vi "Lab3.vi"() -> ()   [LabVIEW 2021]
panel:
  in  "stop":bool
  out "Green 2":bool
  out "Yellow 2":bool
  out "Red 2":bool
  out "Green":bool
  out "Yellow":bool
  out "Red":bool
  out "Is it more than 5?":bool
  out "The number you input is:":string
  in  "Please input a number:":dbl
  in  "To Stop the Operation:":bool
  out "Condition":string
  out "Heater":bool
  out "Air Conditioner":bool
  out "Thermometer":dbl(slide) scale=0.0..100.0
  in  "Temperature":dbl
  # "Traffic Light 1"
  # "Traffic Light 2"
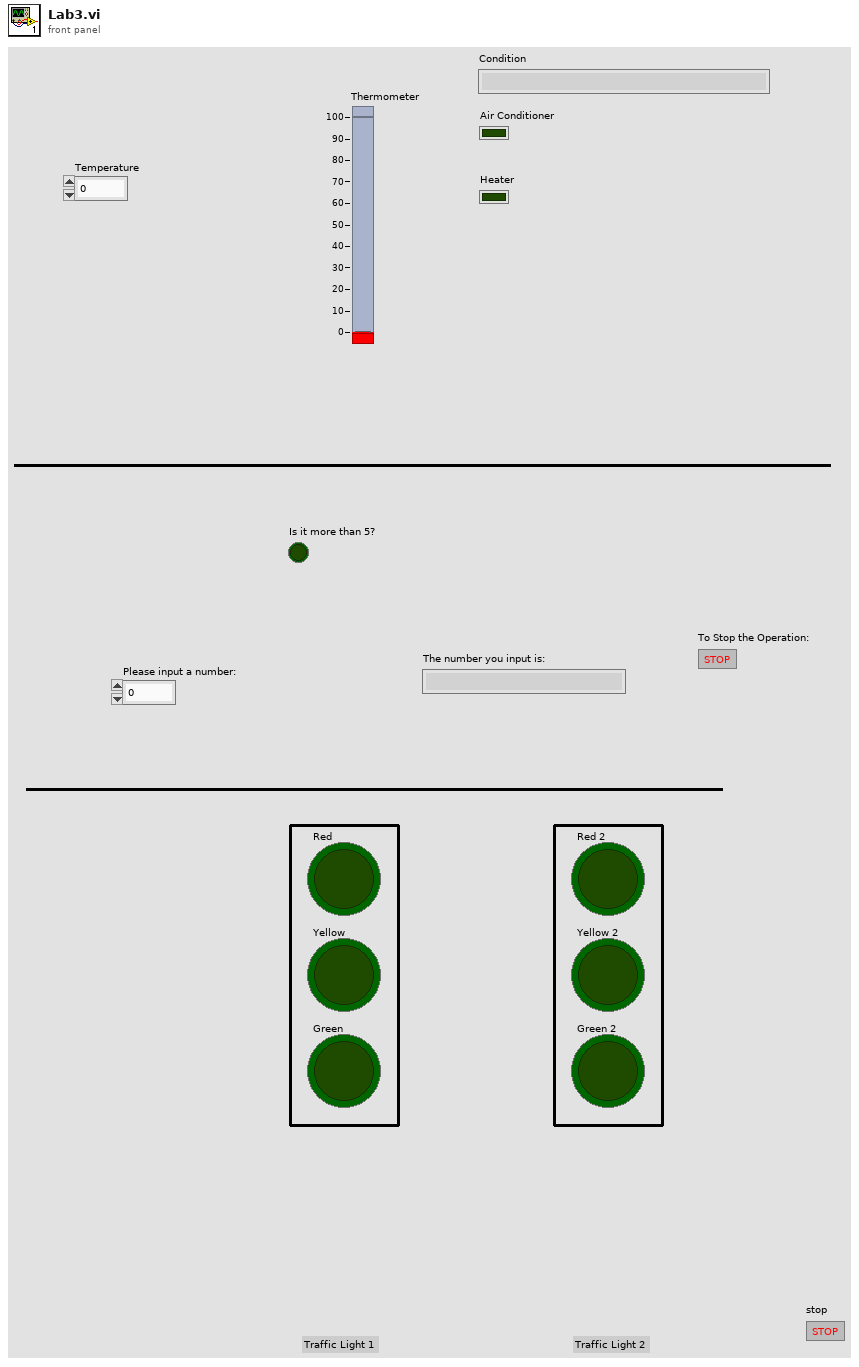
[diagram p1: front panel]
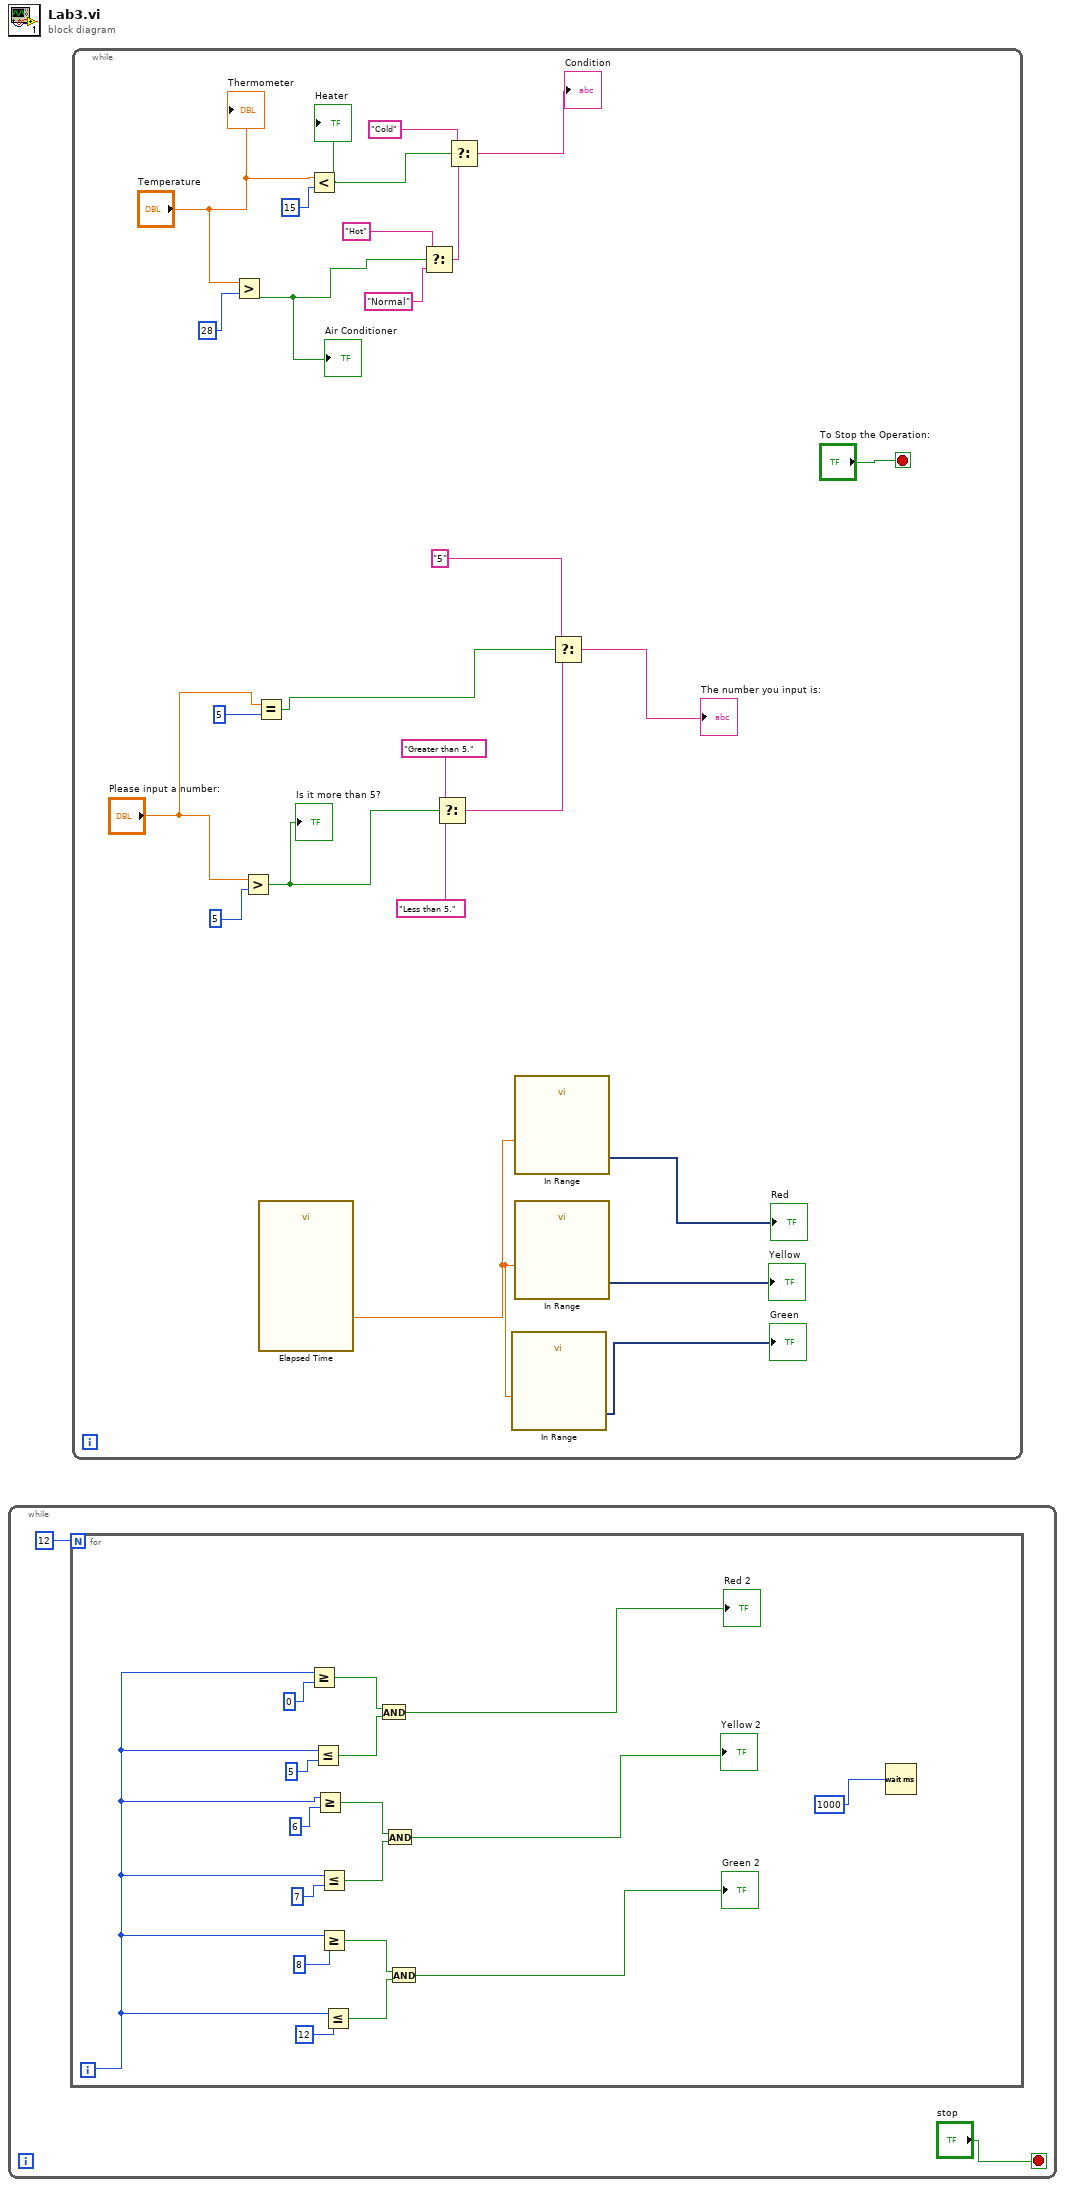
[diagram p0: block diagram]
diagram:
  n1 = while {
    stop <- "stop" stop-if-true
    n2 = for {
      N: 12 -> [_]
      i -> [w4]
      n3 = Greater Or Equal?(x=w4, y=0) -> (x >= y?=w18:bool)
      n4 = Less Or Equal?(x=w4, y=5) -> (x <= y?=w19:bool)
      n5 = Greater Or Equal?(x=w4, y=6) -> (x >= y?=w15:bool)
      n6 = Less Or Equal?(x=w4, y=7) -> (x <= y?=w16:bool)
      n7 = Greater Or Equal?(x=w4, y=8) -> (x >= y?=w12:bool)
      n8 = Less Or Equal?(x=w4, y=12) -> (x <= y?=w13:bool)
      n9 = And(x=w18, y=w19) -> (x .and. y?=→"Red 2":bool)
      n10 = And(x=w15, y=w16) -> (x .and. y?=→"Yellow 2":bool)
      n11 = And(x=w12, y=w13) -> (x .and. y?=→"Green 2":bool)
      n12 = Wait (ms)(milliseconds to wait=1000) -> ()  [unwired: 1 out]
    }
  }
  n13 = while {
    stop <- "To Stop the Operation:" stop-if-true
    n14 = Greater?(x="Temperature", y=28) -> (0:w38:bool)
    "Air Conditioner" <- w38
    n15 = Greater?(x="Please input a number:", y=5) -> (0:w24:bool)
    "Is it more than 5?" <- w24
    n16 = Equal?(x="Please input a number:", y=5) -> (x = y?=w27:bool)
    n17 = call "Elapsed Time"() -> ("Elapsed Time (s)"=w20:dbl)  [unwired: 12 in, 7 out]
    n18 = Less?(x="Temperature", y=15) -> (x < y?=w37:bool)
    "Heater" <- w37
    n19 = Select(t="Hot", s=w38, f="Normal") -> (s? t:f=w40:string)
    n20 = Select(t="Greater than 5.", s=w24, f="Less than 5.") -> (s? t:f=w29:string)
    n21 = Select(t="Cold", s=w37, f=w40) -> (s? t:f=→"Condition":string)
    n22 = call "In Range"("Operand 1"=w20) -> ("Result"=→"Green":dynamicdata)  [unwired: 9 in, 1 out]
    n23 = call "In Range"("Operand 1"=w20) -> ("Result"=→"Red":dynamicdata)  [unwired: 9 in, 1 out]
    n24 = call "In Range"("Operand 1"=w20) -> ("Result"=→"Yellow":dynamicdata)  [unwired: 9 in, 1 out]
    n25 = Select(t="5", s=w27, f=w29) -> (s? t:f=→"The number you input is:":string)
    "Thermometer" <- "Temperature"
  }
